vi "Verify Resolution.vi"(10 "error in":errorcluster) -> (2 "error out":errorcluster, 3 "Abort Launch":bool caption="OK")   [LabVIEW 2023, in "Launcher.lvlib" / "Launcher.lvclass"]
uses:
  Library/Launcher.lvclass
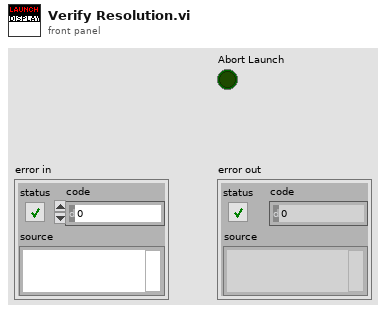
[diagram p1: front panel]
types:
  T1 = typedef "LVRectTypeDef.ctl" = cluster{"Left":i16, "Top":i16, "Right":i16, "Bottom":i16}
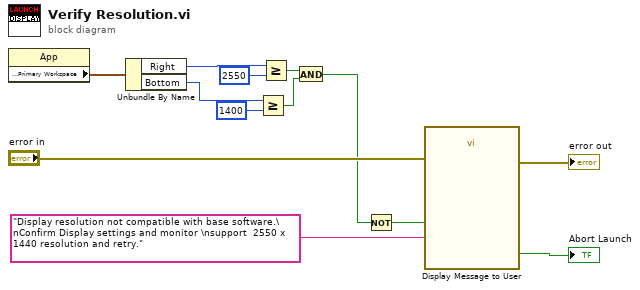
[diagram p0: block diagram]
diagram:
  n1 = property class="App"() -> ("Display:Primary Workspace"=w1:T1)  [unwired: 2 in, 2 out]
  n2 = Unbundle By Name(w1) -> ("Right"=w2:i16, "Bottom"=w3:i16)
  n3 = Greater Or Equal?(x=w3, y=i16 1400) -> (x >= y?=w7:bool)
  n4 = Greater Or Equal?(x=w2, y=i16 2550) -> (x >= y?=w6:bool)
  n5 = And(x=w6, y=w7) -> (x .and. y?=w8:bool)
  n6 = Not(x=w8) -> (.not. x?=w9:bool)
  n7 = call "Display Message to User"("error in (no error)"="error in", "Enable"=w9, "Message"="Display resolution not compatible with base software.\nConfirm Display settings and monitor \nsupport  2550 x 1440 resolution and retry." ("format string")) -> ("error out"=→"error out":errorcluster, "OK"=→"Abort Launch":bool)  [unwired: 7 in]
